vi "WLAN_FrameAnalysis_BothMessages - Modulation Config.vi"(8 "error in (no error)":errorcluster, 9 "SIC Amp":dbl(slide)=1.0 scale=1.0..5.0, 10 "Modulation 2":T1(ring), 11 "input cluster":cluster{"t0":dbl, "dt":dbl, "Y":cdb[]}) -> (0 "error out":errorcluster, 1 "Constellation":cdb[](graph), 2 "Modulation parameter":T2, 3 "SC Bits":i8[](array[numeric]), 4 "Frequency offset":dbl, 5 "SIG valid?":bool, 7 "Base Bits":i8[](array[numeric]))   [LabVIEW 2022 SP3]
panel:
  in  "Point scaler":dbl(slide)=0.8819277108433735 scale=0.8..1.2
  out "Constellation 2":cdb[](graph)
  out "x+y":dbl
  out "Frequency offset(LTF)":dbl
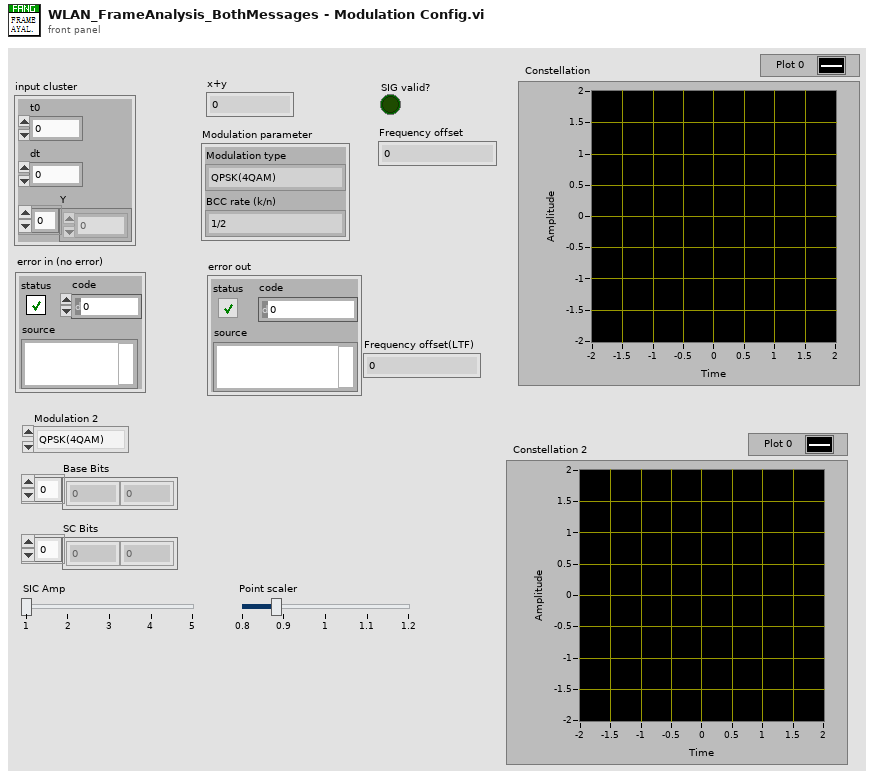
[diagram p1: front panel]
types:
  T1 = enum16{"QPSK(4QAM)", "64QAM", "16QAM", "BPSK", "BPSK Vertical"}
  T2 = cluster{"Modulation type":enum16{"QPSK(4QAM)", "64QAM", "16QAM", "BPSK", "BPSK Vertical"}, "BCC rate (k/n)":enum16{"1/2", "2/3", "3/4"}}
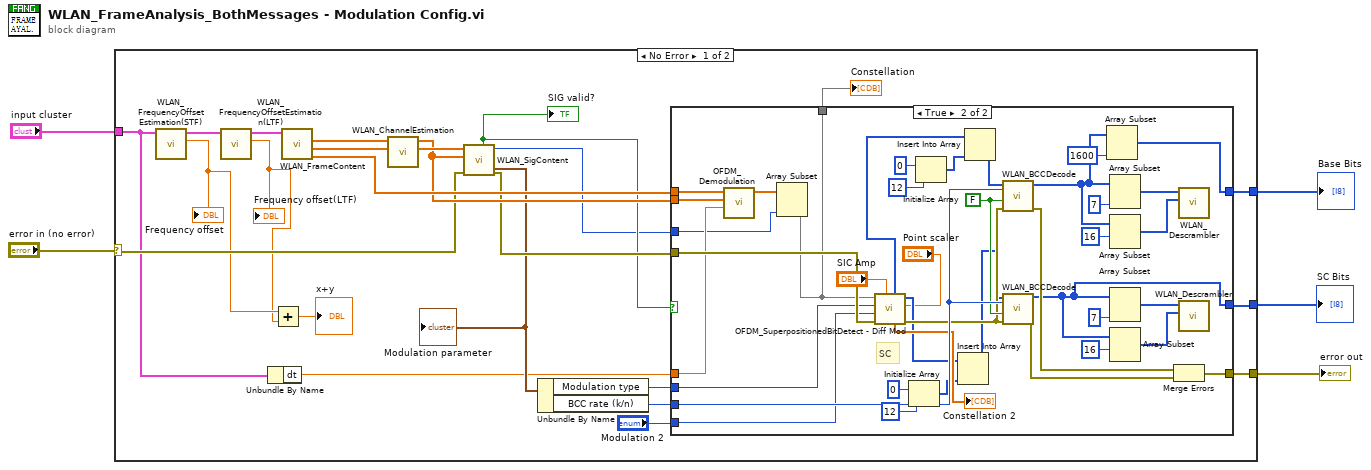
[diagram p0: block diagram]
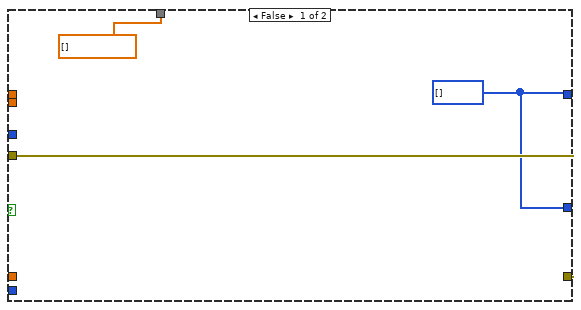
[diagram p2: hidden frame]
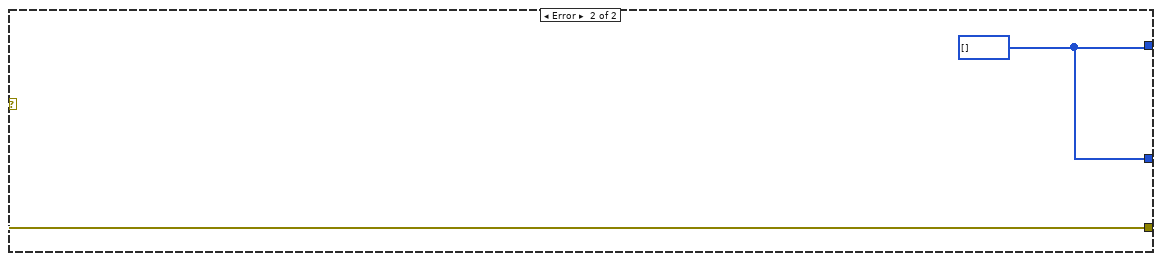
[diagram p3: hidden frame]
diagram:
  n1 = case shown="No Error" "error in (no error)" {
    selector: "error in (no error)" -> [w16 w73]
    tunnel: "input cluster" -> [w10 _]
    tunnel: [w23 w73] -> w4
    tunnel: [w22 w72] -> w3
    tunnel: [w8 w72] -> w1
    frame No Error {
      n2 = call "WLAN_FrequencyOffsetEstimation(STF).vi"("output cluster"=w10) -> ("Frequency offset(STF)"=w14:dbl, "output cluster 2"=w15:cluster{"t0":dbl, "dt":dbl, "Y":cdb[]})  [unwired: 8 in]
      "Frequency offset" <- w14
      n3 = call "WLAN_FrequencyOffsetEstimation(LTF).vi"("input cluster"=w15) -> ("Frequency offset(LTF)"=w13:dbl, "output cluster"=w11:cluster{"t0":dbl, "dt":dbl, "Y":cdb[]})  [unwired: 9 in]
      "Frequency offset(LTF)" <- w13
      n4 = Unbundle By Name(w10) -> ("dt"=w9:dbl)
      n5 = Add(x=w14, y=w13) -> (x+y=→"x+y":dbl)
      n6 = call "WLAN_FrameContent.vi"("Input cluster"=w11) -> ("DATA"=w28:cdb[], "SIG"=w26:cdb[], "LTF"=w27:cdb[])  [unwired: 7 in, 1 out]
      n7 = call "WLAN_ChannelEstimation.vi"("LTF"=w27) -> ("Frequency estimation"=w25:cdb[])  [unwired: 10 in]
      n8 = call "WLAN_SigContent.vi"("error in (no error)"=w16, "Frequency channel estimation"=w25, "SIG"=w26) -> ("error out"=w24:errorcluster, "original bit numbers"=w6:u32, "Modulation parameter"=w21:T2, "SIG valid?"=w17:bool)  [unwired: 3 in, 2 out]
      "Modulation parameter" <- w21
      "SIG valid?" <- w17
      n9 = Unbundle By Name(w21) -> ("Modulation type"=w20:T1, "BCC rate (k/n)"=w19:enum16{"1/2", "2/3", "3/4"})
      n10 = case shown="True" w17 {
        tunnel: w28 -> [_ w71]
        tunnel: [w31 w56] -> w23
        tunnel: w25 -> [_ w69]
        tunnel: w24 -> [w31 w68]
        tunnel: w6 -> [_ w46]
        tunnel: w20 -> [_ w50]
        tunnel: [w29 w47] -> w22
        tunnel: w19 -> [_ w58]
        tunnel: [cdb[] [] w49] -> w18
        tunnel: w9 -> [_ w63]
        tunnel: [w29 w43] -> w8
        tunnel: "Modulation 2" -> [_ w51]
        frame False {
          w29 = i8[] [] ("scrambled bits")
        }
        frame True {
          w57 = FALSE ("need add zeros?")
          # "SC"
          n11 = call "OFDM_Demodulation.vi"("sampling period"=w63, "Frequency channel estimation"=w69, "Input sequence"=w71) -> ("Output sequence"=w70:cdb[])  [unwired: 7 in, 1 out]
          n12 = Array Subset(array=w70, length=w46) -> (w49:cdb[])  [unwired: 1 in]
          n13 = call "OFDM_SuperpositionedBitDetect - Diff Mod.vi"("Input symbols"=w49, "Modulation type"=w50, "Modulation type 2"=w51, "error in (no error)"=w68, "SIC Amp"="SIC Amp", "Point scaler"="Point scaler") -> ("Base Bits"=w38:i8[], "SC Symbols"=→"Constellation 2":cdb[], "SC Bits"=w34:i8[], "error out"=w53:errorcluster)  [unwired: 1 in]
          n14 = Initialize Array(i8 0 ("element"), 12 ("dimension size")) -> (w37:i8[])
          n15 = Initialize Array(i8 0 ("element"), 12 ("dimension size")) -> (w42:i8[])
          n16 = Insert Into Array(array=w34, new element=w37) -> (w33:i8[])  [unwired: 1 in]
          n17 = Insert Into Array(array=w38, new element=w42) -> (w39:i8[])  [unwired: 1 in]
          n18 = call "WLAN_BCCDecode.vi"("error in (no error)"=w53, "need add zeros?"=w57, "BCC rate (k/n)"=w58, "input bit stream"=w39) -> ("error out"=w54:errorcluster, "output bit stream"=w45:i8[])  [unwired: 6 in]
          n19 = call "WLAN_BCCDecode.vi"("error in (no error)"=w53, "need add zeros?"=w57, "BCC rate (k/n)"=w58, "input bit stream"=w33) -> ("error out"=w55:errorcluster, "output bit stream"=w47:i8[])  [unwired: 6 in]
          n20 = Array Subset(array=w45, length=1600) -> (w43:i8[])  [unwired: 1 in]
          n21 = Array Subset(array=w45, length=7) -> (w62:i8[])  [unwired: 1 in]
          n22 = Array Subset(array=w45, index=16) -> (w61:i8[])  [unwired: 1 in]
          n23 = Array Subset(array=w47, length=7) -> (w64:i8[])  [unwired: 1 in]
          n24 = Array Subset(array=w47, index=16) -> (w65:i8[])  [unwired: 1 in]
          n25 = Merge Errors(w54, w55) -> (w56:errorcluster)
          n26 = call "WLAN_Descrambler.vi"("scrambler initial bits"=w62, "data bits"=w61) -> ()  [unwired: 7 in, 1 out]
          n27 = call "WLAN_Descrambler.vi"("scrambler initial bits"=w64, "data bits"=w65) -> ()  [unwired: 7 in, 1 out]
        }
      }
      "Constellation" <- w18
    }
    frame Error {
      w72 = i8[] [] ("scrambled bits")
    }
  }
  "error out" <- w4
  "SC Bits" <- w3
  "Base Bits" <- w1
